vi "xcorr_test_extremas.vi"() -> ()   [LabVIEW 2012]
uses:
  <vilib>/gmath/NI_Gmath.lvlib
panel:
  out "min(x,y)":dbl[](array[numeric])
  out "max(x,y)":dbl[](array[numeric])
  out "Array 3":dbl[](array[numeric])
  out "Array 2":dbl[](array[numeric])
  out "Array":dbl[][](array[numeric])
  in  "data":dbl[][](array[numeric])
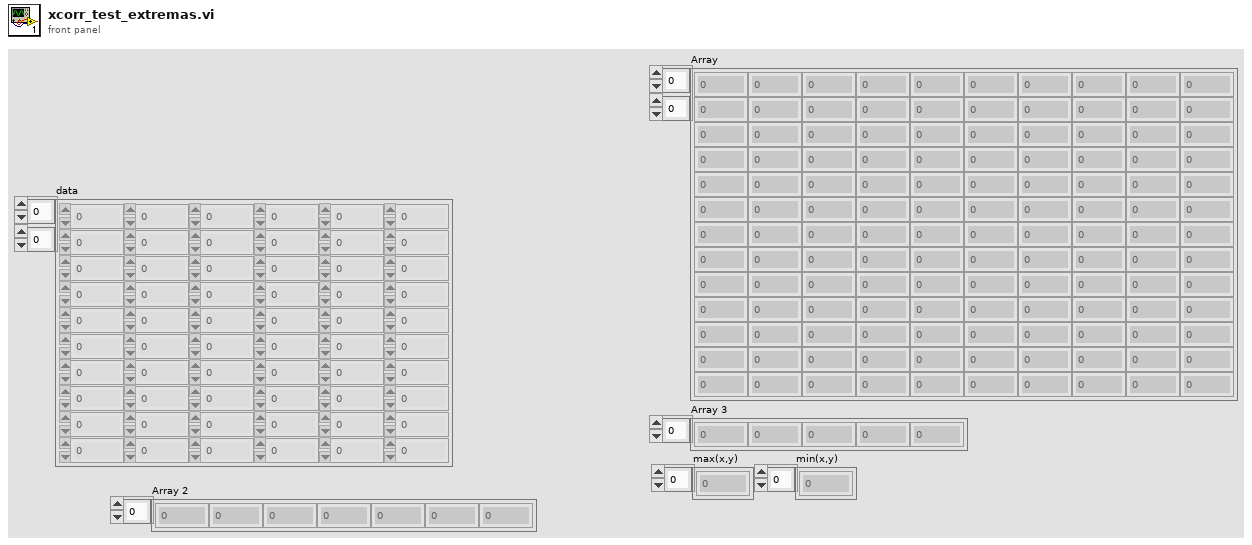
[diagram p1: front panel]
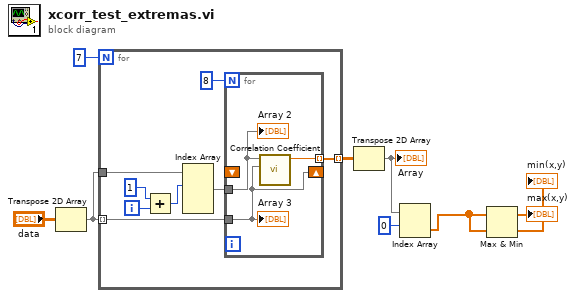
[diagram p0: block diagram]
diagram:
  n1 = Transpose 2D Array(2D array="data") -> (transposed array=w7:dbl[][])
  n2 = for {
    N: 7 -> [_]
    tunnel: [w17] -> w6 mode=indexing
    tunnel: w7 -> [w10] mode=indexing
    tunnel: w7 -> [w13]
    i -> [w16]
    n3 = Add(x=1, y=w16) -> (x+y=w14:i32)
    n4 = Index Array(array=w13, index (row) #1=w14) -> (element #1=w12:dbl[])  [unwired: 3 in, 1 out]
    n5 = for {
      N: 8 -> [_]
      tunnel: [w20] -> w17 mode=indexing
      tunnel: w12 -> [w19]
      tunnel: w10 -> [w18]
      shift-right: [w18] -> _
      shift-left: _ -> [_]
      n6 = call <vilib>:"Correlation Coefficient.vi"("Y"=w18, "X"=w19) -> ("correlation coefficient r"=w20:dbl)  [unwired: 8 in, 1 out]
      "Array 2" <- w19
      "Array 3" <- w18
    }
  }
  n7 = Transpose 2D Array(2D array=w6) -> (transposed array=w5:dbl[][])
  "Array" <- w5
  n8 = Index Array(array=w5, index (row)=0) -> (element=w3:dbl[])  [unwired: 1 in]
  n9 = Max & Min(x=w3, y=w3) -> (max(x,y)=→"max(x,y)":dbl[], min(x,y)=→"min(x,y)":dbl[])
